vi "msecs per Beat.vi"(11 "tt tt tt":u8[](array[numeric]) format="%x") -> (3 "ms per beat":u32)   [LabVIEW 2016]
panel:
  # "Calculated using http://www.somascape.org/midi/tech/mfile.html and http://sites.uci.edu/camp2014/2014/05/19/timing-in-midi-files/"
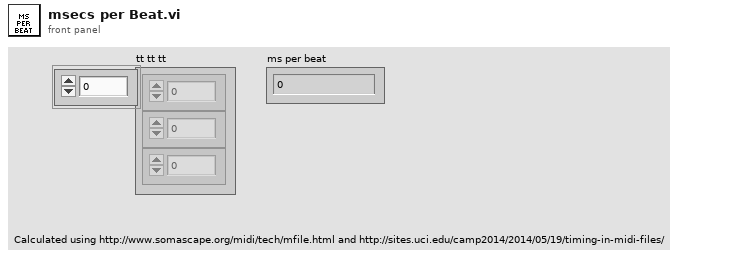
[diagram p1: front panel]
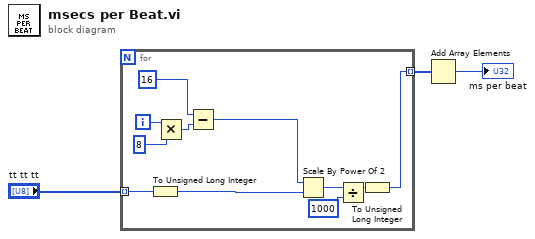
[diagram p0: block diagram]
diagram:
  n1 = for {
    tunnel: "tt tt tt" -> [w14] mode=indexing
    tunnel: [w9] -> w3 mode=indexing
    i -> [w8]
    n2 = To Unsigned Long Integer(number=w14) -> (unsigned 32bit integer=w10:u32)
    n3 = Multiply(x=w8, y=8) -> (x*y=w6:i32)
    n4 = Subtract(x=u32 16, y=w6) -> (x-y=w4:u32)
    n5 = Scale By Power Of 2(n=w4, x=w10) -> (x*2^n=w13:u32)
    n6 = Divide(x=w13, y=u32 1000) -> (x/y=w12:dbl)
    n7 = To Unsigned Long Integer(number=w12) -> (unsigned 32bit integer=w9:u32)
  }
  n8 = Add Array Elements(numeric array=w3) -> (sum=→"ms per beat":u32)
